vi "From Standard Sequence.vi"(8 "error in (no error)":errorcluster, 10 "Standard Sequence":string[][](array[string])=[["Simple", "", "", ""], ["Wait", "1000", "", ""], ["Update", "Boolean result 0", "Boolean", "True"], ["Wait ", "1000", "", ""], ["Update", "Boolean result 0", "Boolean", "False"]]) -> (0 "error out":errorcluster, 3 "Sequence Config.lvclass":refnum<class "Sequence Config.lvclass">)   [LabVIEW 2015, in "Sequence Config.lvclass"]
uses:
  Sequence Config.lvclass
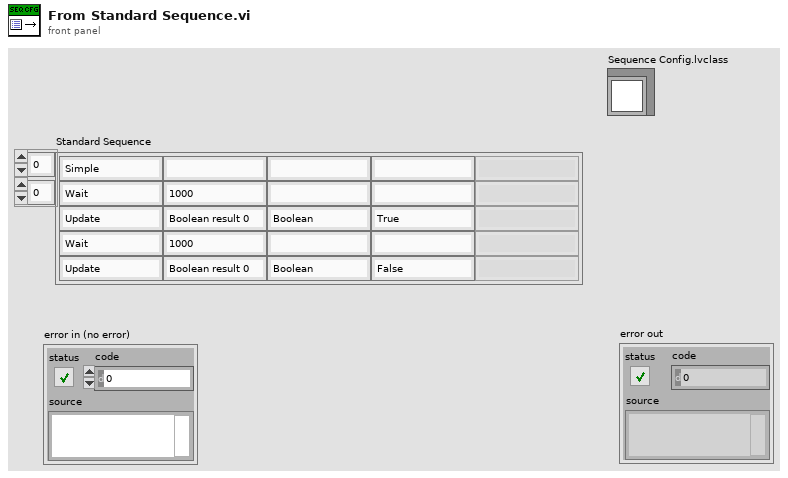
[diagram p1: front panel]
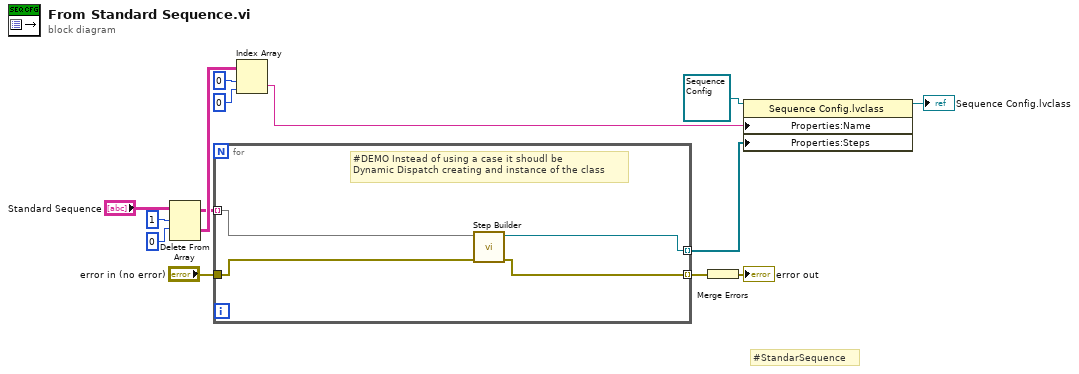
[diagram p0: block diagram]
diagram:
  # "#StandarSequence"
  n1 = Delete From Array(array="Standard Sequence", length=1, index (row)=0) -> (deleted portion=w11:string[][], array with subset deleted=w9:string[][])  [unwired: 1 in]
  n2 = for {
    tunnel: w9 -> [w18] mode=indexing
    tunnel: "error in (no error)" -> [w16]
    tunnel: [w17] -> w3 mode=indexing
    tunnel: [w15] -> w2 mode=indexing
    # "#DEMO Instead of using a case it shoudl be\nDynamic Dispatch creating and instance of the class"
    n3 = call "Step Builder.vi"("error in (no error)"=w16, "Standard Sequence"=w18) -> ("error out"=w15:errorcluster, "Step Config out"=w17:refnum<class "Step Config.lvclass">)  [unwired: 8 in]
  }
  n4 = Index Array(array=w11, index (row)=0 ("index"), index (col)=0 ("disabled index (col)")) -> (element=w4:string)
  n5 = Merge Errors(w2) -> (→"error out":errorcluster)
  n6 = property class="Sequence Config.lvclass"(reference=refnum<class "Sequence Config.lvclass"> refnum ("Sequence Config.lvclass"), "Properties:Name"=w4, "Properties:Steps"=w3) -> (reference out=→"Sequence Config.lvclass":refnum<class "Sequence Config.lvclass">)  [unwired: 1 in, 1 out]
